vi "Frame Page.vi"(8 "error in (no error)":errorcluster, 11 "Node Ptr":T1 format="%.0x") -> (0 "error out":errorcluster)   [LabVIEW 2019, in "Ghost Bus Addon System Explorer.lvlib"]
uses:
  Ghost Bus Addon System Explorer.lvlib
  <vilib>/NI VeriStand/Custom Device API/Custom Device API.lvlib
  Addon Shared/SubVIs/GUID Lookup.vi
  Addon Shared/Ghost Bus Addon Shared.lvlib
  <vilib>/NI VeriStand/Custom Device API/Custom Device Item Ref.ctl
panel:
  in  "Description":string
  out "Frame ID":u32 format="%.0x"
  in  "Custom Device Settings":cluster{"Section Name":string}={"Section Name"="Frame Settings"}
  out "Name":string
  in  "SHDocVw.IWebBrowser2":refnum<k7>(container)
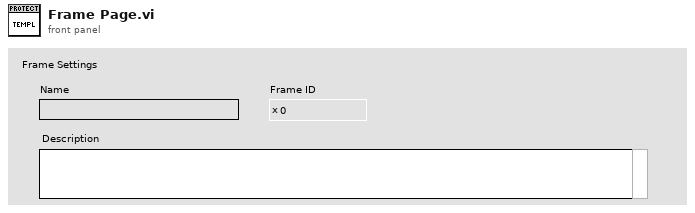
[diagram p1: front panel]
types:
  T1 = typedef "Custom Device API.lvlib/Custom Device Item Ref.ctl" = u64
  T2 = typedef "Frame Settings.ctl" = cluster{"ID":u32}
  T3 = typedef "Custom Device API.lvlib/Custom Device Item Info.ctl" = cluster{"Name":string, "Is Channel":bool, "GUID":string, "Is Waveform":bool}
  T4 = typedef "Custom Device API.lvlib/Custom Device Commands.ctl" = enum16{"Default", "Item renamed", "Shutdown", "Dynamic button pressed"}
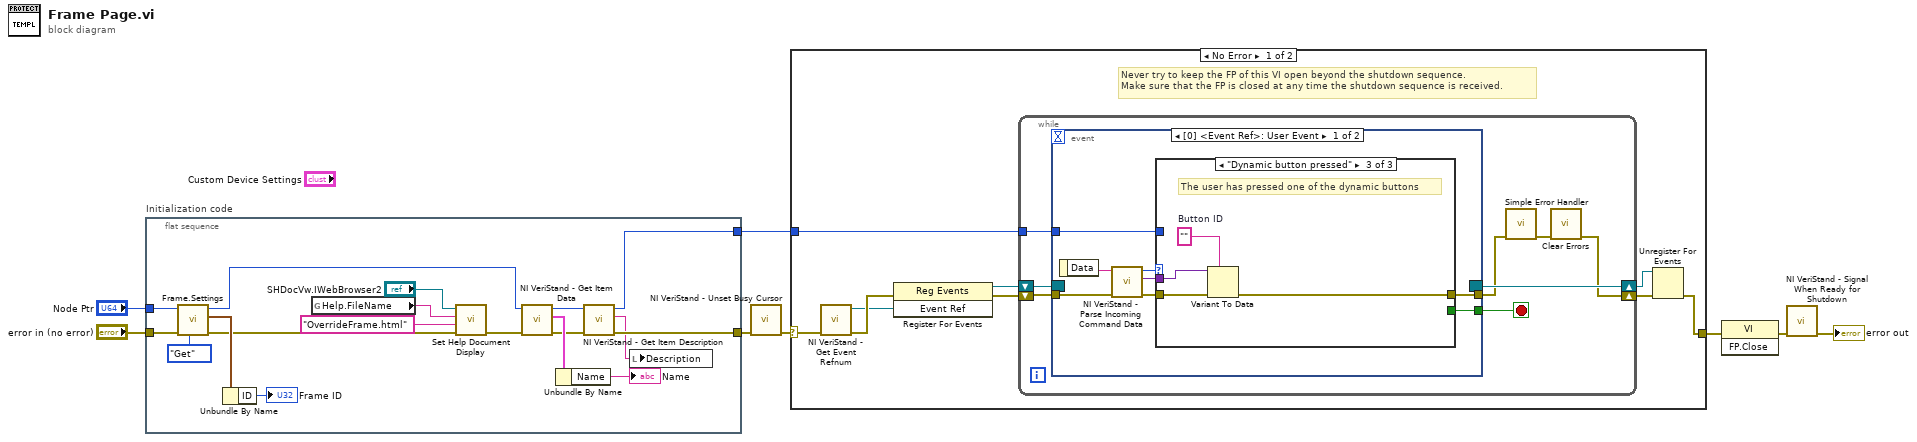
[diagram p0: block diagram]
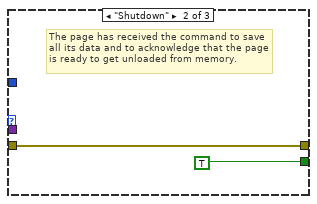
[diagram p3: hidden frame]
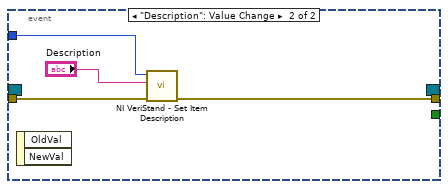
[diagram p4: hidden frame]
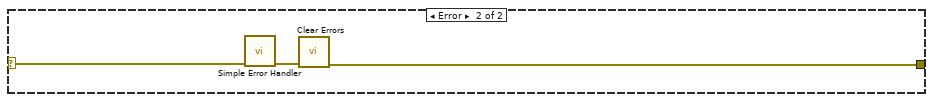
[diagram p5: hidden frame]
diagram:
  n1 = flat-sequence "Initialization code" {
    tunnel: "error in (no error)" -> [w15]
    tunnel: "Node Ptr" -> [w14]
    tunnel: [w21] -> w3
    tunnel: [w19] -> w1
    frame #0 {
      n2 = call "Frame.Settings.vi"("Action"=enum8{"Get", "Set"}."Get", "error in (no error)"=w15, "Item Ref in"=w14) -> ("error out"=w11:errorcluster, "Frame.Settings"=w17:T2, "Item Ref out"=w9:T1)  [unwired: 6 in]
      n3 = Unbundle By Name(w17) -> ("ID"=→"Frame ID":u32)
      n4 = global read "GUID Lookup.vi" "Help.FileName"() -> (w12:string)
      n5 = call "Set Help Document Display.vi"("error in (no error)"=w11, "HTML File"="OverrideFrame.html", "Main CHM File"=w12, "SHDocVw.IWebBrowser2"="SHDocVw.IWebBrowser2") -> ("error out"=w10:errorcluster)  [unwired: 7 in]
      n6 = call <vilib>:"NI VeriStand - Get Item Data.vi"("error in (no error)"=w10, "Item Ref in"=w9) -> ("error out"=w22:errorcluster, "Item Info"=w24:T3, "Item Ref out"=w20:T1)  [unwired: 7 out]
      n7 = Unbundle By Name(w24) -> ("Name"=→"Name":string)
      n8 = call <vilib>:"NI VeriStand - Get Item Description.vi"("error in (no error)"=w22, "Item Ref in"=w20) -> ("error out"=w21:errorcluster, "Description"=w18:string, "Item Ref out"=w19:T1)  [unwired: 7 out]
      n9 = local write "Description"(w18) -> ()
    }
  }
  n10 = call <vilib>:"NI VeriStand - Unset Busy Cursor.vi"("error in (no error)"=w3) -> ("error out"=w5:errorcluster)  [unwired: 10 out]
  n11 = case shown="No Error" w5 {
    selector: w5 -> [w27 w65]
    tunnel: [w32 w63] -> w8
    tunnel: w1 -> [w28 _]
    frame No Error {
      # "Never try to keep the FP of this VI open beyond the shutdown sequence.\nMake sure that the FP is closed at any time the shutdown sequence is received."
      n12 = call <vilib>:"NI VeriStand - Get Event Refnum.vi"("error in (no error)"=w27) -> ("error out"=w35:errorcluster, "Event Ref"=w31:refnum<user-event>)  [unwired: 9 out]
      n13 = register-events(error in=w35, w31) -> (reference out=w29:refnum<event-registration>, error out=w30:errorcluster)  [unwired: 1 in]
      n14 = while {
        tunnel: w28 -> [w39]
        shift-right: [w36] -> w33
        shift-left: w30 -> [w42]
        shift-right: [w43] -> w34
        shift-left: w29 -> [w41]
        stop <- w40 stop-if-true
        n15 = event shown="[0] <Event Ref>: User Event" {
          selector: w41 -> [_ _]
          dyn-events: [_ _] -> w43
          timeout: _ -> [_ _]
          tunnel: w42 -> [w51 w62]
          tunnel: [w47 _] -> w40
          tunnel: [w46 w61] -> w38
          tunnel: w39 -> [w45 w60]
          event User Event {
            n16 = event-data() -> ("Data"=w50:string)  [unwired: 1 out]
            n17 = call <vilib>:"NI VeriStand - Parse Incoming Command Data.vi"("error in (no error)"=w51, "Incoming data"=w50) -> ("error out"=w49:errorcluster, "Outgoing data"=w44:variant, "Action"=w48:T4)  [unwired: 7 out]
            n18 = case shown="\"Dynamic button pressed\"" w48 {
              tunnel: w49 -> [w52 w53 w58]
              tunnel: [_ TRUE _] -> w47
              tunnel: [w52 w53 w55] -> w46
              tunnel: w45 -> [_ _ _]
              tunnel: w44 -> [_ _ w57]
              frame "Default", Default {
              }
              frame "Shutdown" {
                # "The page has received the command to save all its data and to acknowledge that the page is ready to get unloaded from memory."
              }
              frame "Dynamic button pressed" {
                w56 = ""  # Button ID
                # "The user has pressed one of the dynamic buttons"
                n19 = Variant To Data(error in=w58, type=w56, Variant=w57) -> (error out=w55:errorcluster)  [unwired: 1 out]
              }
            }
          }
          event "Description": Value Change {
            n20 = event-data() -> ()  [unwired: 3 out]
            n21 = call <vilib>:"NI VeriStand - Set Item Description.vi"("error in (no error)"=w62, "Description"="Description", "Item Ref in"=w60) -> ("error out"=w61:errorcluster)  [unwired: 8 out]
          }
        }
        n22 = call <vilib>:"Simple Error Handler.vi"("error in (no error)"=w38) -> ("error out"=w37:errorcluster)  [unwired: 1 in, 7 out]
        n23 = call <vilib>:"Clear Errors.vi"("error in (no error)"=w37) -> ("error out"=w36:errorcluster)  [unwired: 1 in, 5 out]
      }
      n24 = Unregister For Events(event registration refnum=w34, error in=w33) -> (error out=w32:errorcluster)
    }
    frame Error {
      n25 = call <vilib>:"Simple Error Handler.vi"("error in (no error)"=w65) -> ("error out"=w64:errorcluster)  [unwired: 1 in, 7 out]
      n26 = call <vilib>:"Clear Errors.vi"("error in (no error)"=w64) -> ("error out"=w63:errorcluster)  [unwired: 1 in, 5 out]
    }
  }
  n27 = invoke class="VI" method="FP.Close"(error in=w8) -> (error out=w7:errorcluster)  [unwired: 2 in, 2 out]
  n28 = call <vilib>:"NI VeriStand - Signal When Ready for Shutdown.vi"("error in (no error)"=w7) -> ("error out"=→"error out":errorcluster)  [unwired: 10 out]
